vi "Parse and Format Program Freq Table String for Downlink.vi"(10 "Input String":string) -> (2 "Output String":string)   [LabVIEW 2010]
doc: "This VI parses the ProgramFreqTable entries from the iput string and formats the data for downlink."
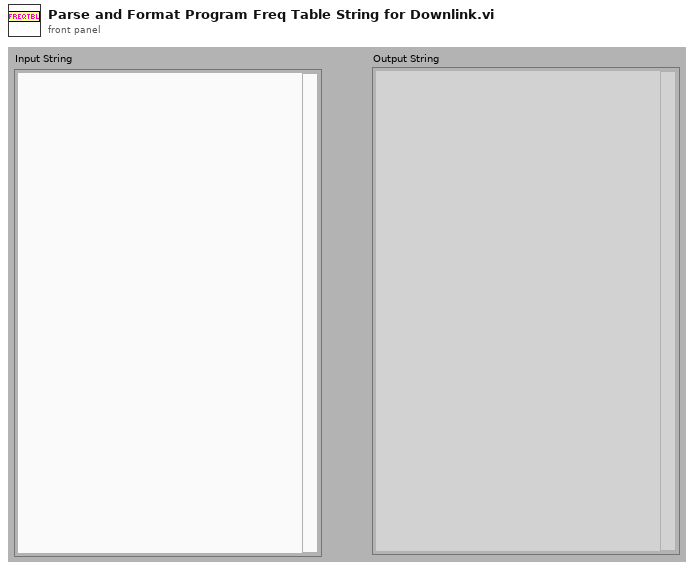
[diagram p1: front panel]
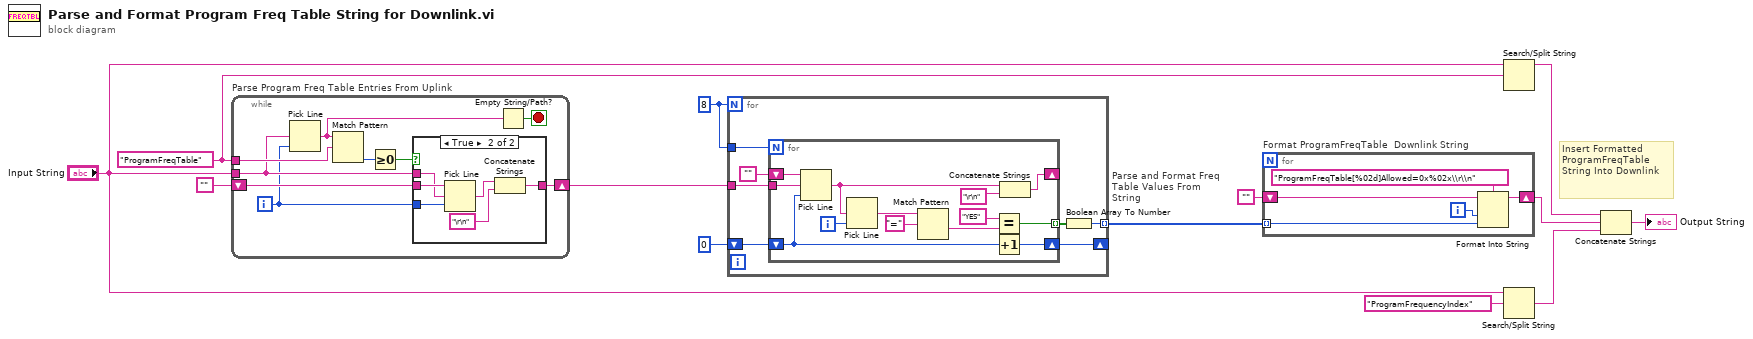
[diagram p0: block diagram]
diagram:
  w1 = "ProgramFreqTable" ("regular expression")
  w3 = 8
  # "Insert Formatted ProgramFreqTable String Into Downlink"
  n1 = while "Parse Program Freq Table Entries From Uplink" {
    shift-right: [w22] -> w5
    shift-left: "" -> [w21]
    tunnel: "Input String" -> [w15]
    tunnel: w1 -> [w16]
    i -> [w14]
    stop <- w20 stop-if-true
    n2 = Pick Line(multi-line string=w15, line index=w14) -> (output string=w17:string)  [unwired: 1 in]
    n3 = Match Pattern(string=w17, regular expression=w16) -> (offset past match=w18:i32)  [unwired: 1 in, 3 out]
    n4 = Greater Or Equal To 0?(x=w18) -> (x >= 0?=w19:bool)
    n5 = case shown="True" w19 {
      tunnel: w14 -> [_ w29]
      tunnel: [w23 w26] -> w22
      tunnel: w21 -> [w23 w25]
      tunnel: w15 -> [_ w24]
      frame False {
      }
      frame True {
        n6 = Pick Line(string ("")=w25, multi-line string=w24, line index=w29) -> (output string=w27:string)
        n7 = Concatenate Strings(w27, "\r\n" ("string")) -> (w26:string)
      }
    }
    n8 = Empty String/Path?(string/path=w17) -> (empty?=w20:bool)
  }
  n9 = for "Parse and Format Freq Table Values From String" {
    N: w3 -> [_]
    tunnel: w5 -> [w32]
    tunnel: w3 -> [w34]
    tunnel: [w35] -> w6 mode=indexing
    shift-right: [w30] -> _
    shift-left: 0 -> [w31]
    n10 = for {
      N: w34 -> [_]
      shift-right: [w47] -> _
      shift-left: "" -> [w49]
      tunnel: [w44] -> w36 mode=indexing
      tunnel: w32 -> [w40]
      shift-right: [w38] -> w30
      shift-left: w31 -> [w39]
      i -> [w37]
      n11 = Pick Line(string ("")=w49, multi-line string=w40, line index=w39) -> (output string=w41:string)
      n12 = Pick Line(multi-line string=w41, line index=w37) -> (output string=w42:string)  [unwired: 1 in]
      n13 = Match Pattern(string=w42, regular expression="=" ("search string/char (-)")) -> (after substring=w43:string)  [unwired: 1 in, 3 out]
      n14 = Equal?(x="YES", y=w43) -> (x = y?=w44:bool)
      n15 = Increment(x=w39) -> (x+1=w38:i32)
      n16 = Concatenate Strings(w41, "\r\n" ("string")) -> (w47:string)
    }
    n17 = Boolean Array To Number(Boolean array=w36) -> (number=w35:u32)
  }
  n18 = for "Format ProgramFreqTable  Downlink String" {
    shift-right: [w52] -> w12
    shift-left: "" -> [w54]
    tunnel: w6 -> [w51] mode=indexing
    i -> [w50]
    n19 = Format Into String(format string="ProgramFreqTable[%02d]Allowed=0x%02x\\r\\n", initial string=w54, w50, w51) -> (resulting string=w52:string)  [unwired: 1 in, 1 out]
  }
  n20 = Search/Split String(string="Input String", search string/char (-)=w1) -> (substring before match=w8:string)  [unwired: 1 in, 2 out]
  n21 = Search/Split String(string="Input String", search string/char (-)="ProgramFrequencyIndex") -> (match + rest of string=w11:string)  [unwired: 1 in, 2 out]
  n22 = Concatenate Strings(w8, w12, w11) -> (→"Output String":string)
